vi "svfa_Tone Estimation Subroutine G(f) (magnitude).vi"(4 "N (window length)":i32=512, 5 "window":T1(ring), 6 "frequency":dbl format="%.5e", 7 "three fingers":cluster{"f0":dbl, "df":dbl, "spectrum":dbl[]}={"f0"=0.0, "df"=1.0, "spectrum"=[]} {"spectrum" format="%.2f"; "df" format="%.2f"; "f0" format="%.2f"}) -> (2 "Amplitude":dbl format="%.2f", 3 "G(f)":dbl format="%.2e")   [LabVIEW 2017]
doc: "This is the actual function involved in the Newton-Raphson's root finding loop.\nG(f) is the function to be evaluated. for each iteration, amplitude and phase are also computed."
uses:
  <vilib>/addons/_NISVFA/_Spectrum Processing/subVIs/svfa_Window Frequency Response (double array).vi
  <vilib>/addons/_NISVFA/_Spectrum Processing/subVIs/svfa_Rect Window Frequency Response.vi
  <vilib>/addons/_NISVFA/_Spectrum Processing/subVIs/svfa_Cosine Window Coefficients.vi
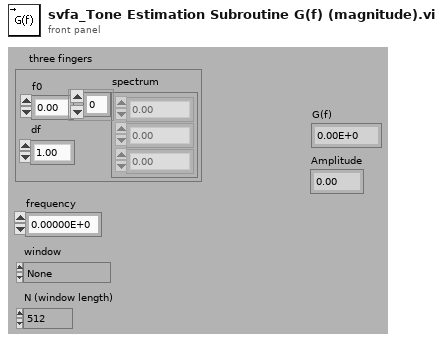
[diagram p1: front panel]
types:
  T1 = enum16{"None ", "Hanning", "Hamming", "Blackman-Harris", "Exact Blackman", "Blackman", "Flat Top", "4 Term B-Harris ", "7 Term B-Harris", "Low Sidelobe"}
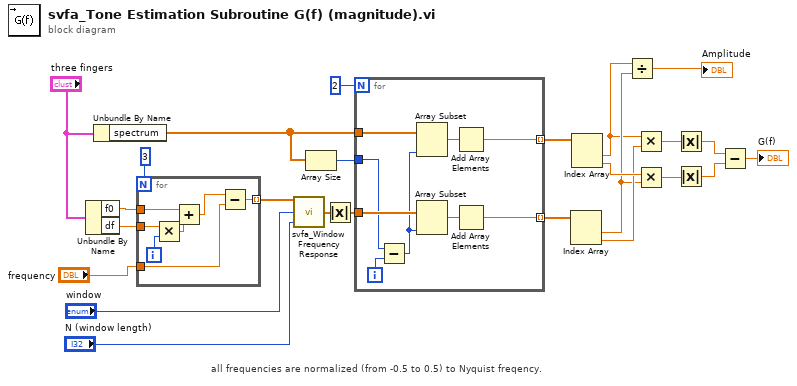
[diagram p0: block diagram]
diagram:
  # "all frequencies are normalized (from -0.5 to 0.5) to Nyquist freqency."
  n1 = Unbundle By Name("three fingers") -> ("f0"=w2:dbl, "df"=w1:dbl)
  n2 = Unbundle By Name("three fingers") -> ("spectrum"=w4:dbl[])
  n3 = for {
    N: 3 -> [_]
    tunnel: w2 -> [w32]
    tunnel: w1 -> [w29]
    tunnel: "frequency" -> [w27]
    tunnel: [w26] -> w21 mode=indexing
    i -> [w30]
    n4 = Multiply(x=w29, y=w30) -> (x*y=w31:dbl)
    n5 = Add(x=w32, y=w31) -> (x+y=w28:dbl)
    n6 = Subtract(x=w28, y=w27) -> (x-y=w26:dbl)
  }
  n7 = call-poly <vilib>:"svfa_Window Frequency Response.vi"("N (window length)"="N (window length)", "window"="window", "f(normalized)"=w21) -> ("H(f)"=w19:cdb[])
  n8 = Array Size(array=w4) -> (size(s)=w13:i32)
  n9 = Absolute Value(x=w19) -> (abs(x)=w7:dbl[])
  n10 = for {
    N: 2 -> [_]
    tunnel: w4 -> [w41]
    tunnel: w7 -> [w40]
    tunnel: [w34] -> w17 mode=indexing
    tunnel: [w33] -> w16 mode=indexing
    tunnel: w13 -> [w37]
    i -> [w39]
    n11 = Subtract(x=w37, y=w39) -> (x-y=w38:i32)
    n12 = Array Subset(array=w41, length=w38) -> (w36:dbl[])  [unwired: 1 in]
    n13 = Array Subset(array=w40, length=w38) -> (w35:dbl[])  [unwired: 1 in]
    n14 = Add Array Elements(numeric array=w36) -> (sum=w34:dbl)
    n15 = Add Array Elements(numeric array=w35) -> (sum=w33:dbl)
  }
  n16 = Index Array(array=w16) -> (element #1=w10:dbl, element #2=w11:dbl)  [unwired: 2 in]
  n17 = Index Array(array=w17) -> (element #1=w9:dbl, element #2=w12:dbl)  [unwired: 2 in]
  n18 = Divide(x=w9, y=w10) -> (x/y=→"Amplitude":dbl)
  n19 = Multiply(x=w9, y=w11) -> (x*y=w15:dbl)
  n20 = Multiply(x=w12, y=w10) -> (x*y=w14:dbl)
  n21 = Absolute Value(x=w15) -> (abs(x)=w24:dbl)
  n22 = Absolute Value(x=w14) -> (abs(x)=w23:dbl)
  n23 = Subtract(x=w24, y=w23) -> (x-y=→"G(f)":dbl)
